vi "XYZStage-Set max speed command (ver 2).vi"(8 "Error In":errorcluster, 10 "XYZ Stage data":T1={"Command"=enum."Initialize", "Channel"="Z", "X"=0.0, "Y"=0.0, "Z"=0.0, "Speed"=0, "Zero"=FALSE, "Use acknowledgement?"=TRUE} {"Speed" format="Speed= %.0f"; "Z" format="Z= %#_g"; "Y" format="Y= %#_g"; "X" format="X= %#_g"}, 11 "XYZ Stage Control in":refnum<class "XYZ Stage Control.lvclass">) -> (0 "Error Out":errorcluster, 3 "XYZ Stage Control out":refnum<class "XYZ Stage Control.lvclass">)   [LabVIEW 2020]
uses:
  Typedefs/XYZ stage data.ctl
  Typedefs/XYZ stage states.ctl
  Typedefs/XYZ channel ring.ctl
  XYZ Stage Control/XYZ Stage Control.lvclass
  XYZ Stage Control/typedefs/XYZ_position_input.ctl
  XYZ Stage Control/typedefs/XYZ axes.ctl
  Typedefs/XYZ_coordinates.ctl
  Typedefs/Command acknowledgment states.ctl
panel:
  out "read string":string
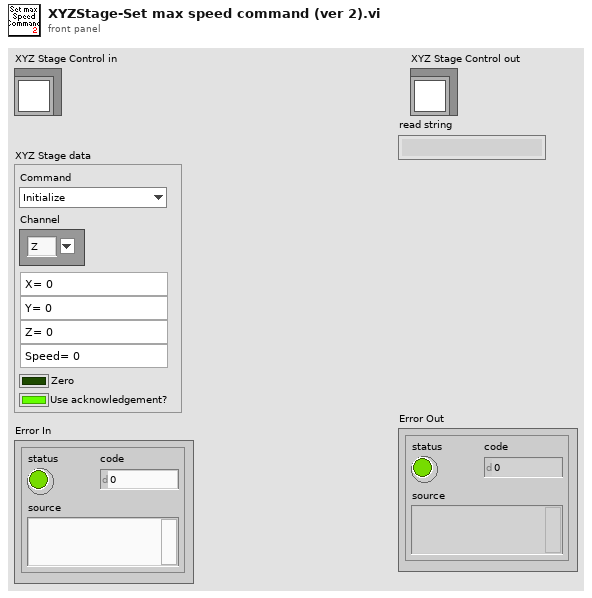
[diagram p1: front panel]
types:
  T1 = typedef "XYZ stage data.ctl" = cluster{"Command":T2, "Channel":T3, "X":sgl, "Y":sgl, "Z":sgl, "Speed":i32, "Zero":bool, "Use acknowledgement?":bool}
  T2 = typedef "XYZ stage states.ctl" = enum16{"Dequeue", "Initialize", "Read Position", "Read Speed Setting", "Move", "Set Max Speed", "Reset Axis", "Stop all movement"}
  T3 = typedef "XYZ channel ring.ctl" = string
  T4 = typedef "XYZ_position_input.ctl" = cluster{"Speed":i32, "Z Limit (um+/-)":sgl, "Axes":T5, "XYZ Coordinates":T6}
  T5 = typedef "XYZ axes.ctl" = string
  T6 = typedef "XYZ_coordinates.ctl" = cluster{"X":sgl, "Y":sgl, "Z":sgl}
  T7 = typedef "Command acknowledgment states.ctl" = enum16{"Acknowledge", "Wait for acknowledgment", "Release queue"}
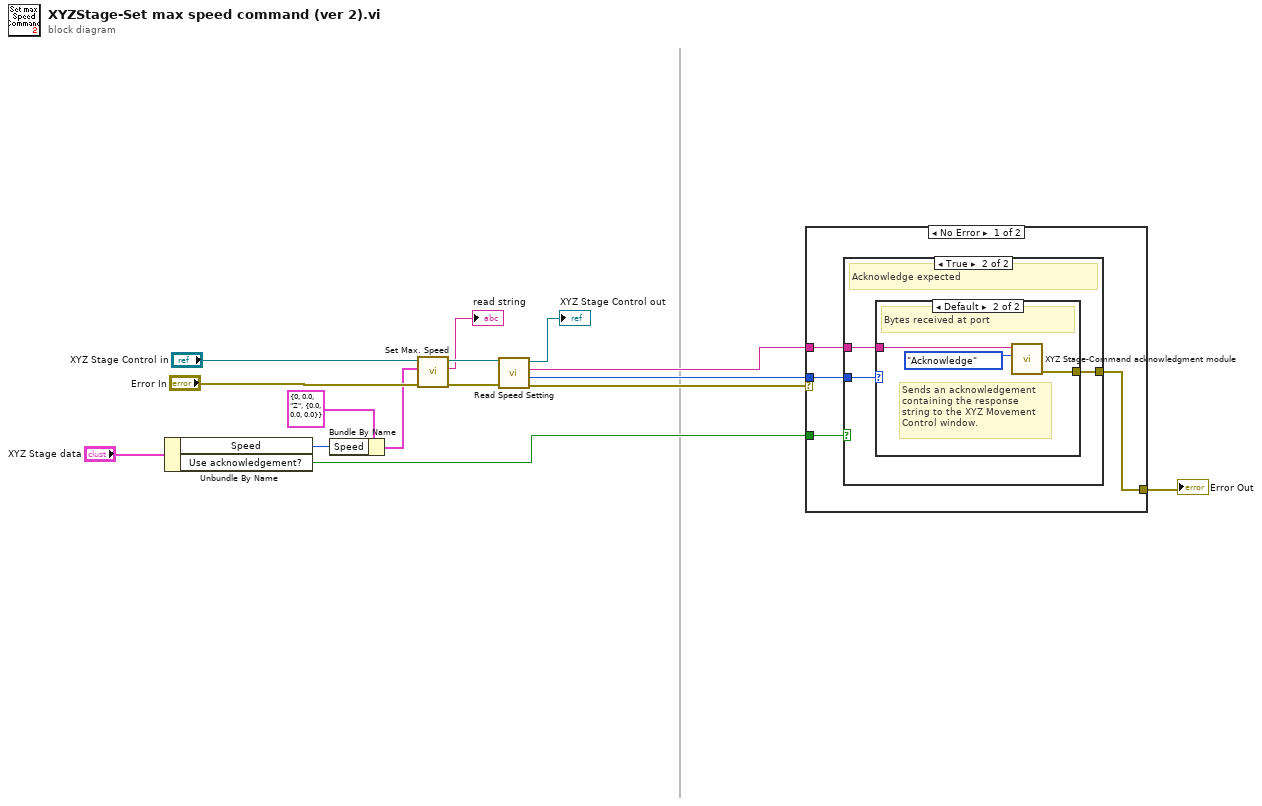
[diagram p0: block diagram]
diagram:
  n1 = Unbundle By Name("XYZ Stage data") -> ("Speed"=w12:i32, "Use acknowledgement?"=w1:bool)
  n2 = Bundle By Name(cluster=T4 {"Speed"=0, "Z Limit (um+/-)"=0.0, "Axes"="Z", "XYZ Coordinates"={"X"=0.0, "Y"=0.0, "Z"=0.0}} ("XYZ Position Input"), "Speed"=w12) -> (w10:T4)
  n3 = call-dynamic "Set Max. Speed.vi"("error in (no error)"="Error In", "XYZ Position Input"=w10, "XYZ Stage Control in"="XYZ Stage Control in") -> ("error out"=w9:errorcluster, "read string"=→"read string":string, "XYZ Stage Control out"=w8:refnum<class "XYZ Stage Control.lvclass">)  [unwired: 6 in]
  n4 = call-dynamic "Read Speed Setting.vi"("error in (no error)"=w9, "XYZ Stage Control in"=w8) -> ("error out"=w3:errorcluster, "bytes read"=w4:u32, "Speed Setting"=w5:string, "XYZ Stage Control out"=→"XYZ Stage Control out":refnum<class "XYZ Stage Control.lvclass">)  [unwired: 6 in]
  n5 = case shown="No Error" w3 {
    selector: w3 -> [_ w26]
    tunnel: w1 -> [w19 _]
    tunnel: w5 -> [w18 _]
    tunnel: [w17 w26] -> w2
    tunnel: w4 -> [w16 _]
    frame No Error {
      n6 = case shown="True" w19 {
        tunnel: w18 -> [_ w22]
        tunnel: [_ w21] -> w17
        tunnel: w16 -> [_ w20]
        frame False {
          # "No acknowledgement expected"
        }
        frame True {
          # "Acknowledge expected"
          n7 = case shown="Default" w20 {
            tunnel: w22 -> [_ w24]
            tunnel: [_ w23] -> w21
            frame 0 {
              # "No data at port"
            }
            frame Default {
              # "Sends an acknowledgement containing the response string to the XYZ Movement Control window."
              # "Bytes received at port"
              n8 = call "XYZ Stage-Command acknowledgment module.vi"("State"=Command_acknowledgment_states."Acknowledge", "Acknowledgement Message in"=w24) -> ("error out"=w23:errorcluster)  [unwired: 7 in, 2 out]
            }
          }
        }
      }
    }
    frame Error {
    }
  }
  "Error Out" <- w2
